vi "RPC Method Template.vi"(8 "error in (no error)":errorcluster, 11 "OOP Server in":refnum<class "OOP Query Server.lvclass">) -> (0 "error out":errorcluster)   [LabVIEW 2019, in "OOP Query Server.lvlib" / "OOP Query Server.lvclass"]
uses:
  OOP Query Server.lvclass
  OOP Query Server.lvclass/OOP Query Server.ctl
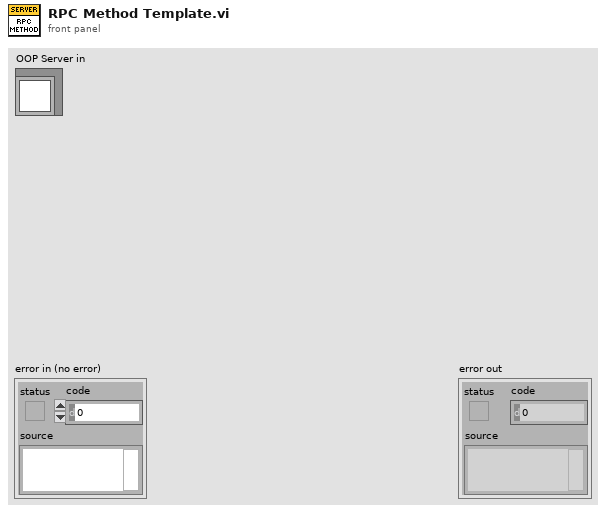
[diagram p1: front panel]
types:
  T1 = typedef "OOP Query Server.lvlib/OOP Query Server.lvclass/Server Internal UEs.ctl" = cluster{"Invoke Internal UE":refnum<user-event>, "Query Internal UE":refnum<user-event>, "Register Internal UE":refnum<user-event>}
  T2 = typedef "OOP Query Server.lvlib/OOP Query Server.lvclass/Server gRPC UEs.ctl" = cluster{"Invoke gRPC UE":refnum<user-event>, "Query gRPC UE":refnum<user-event>, "Register gRPC UE":refnum<user-event>}
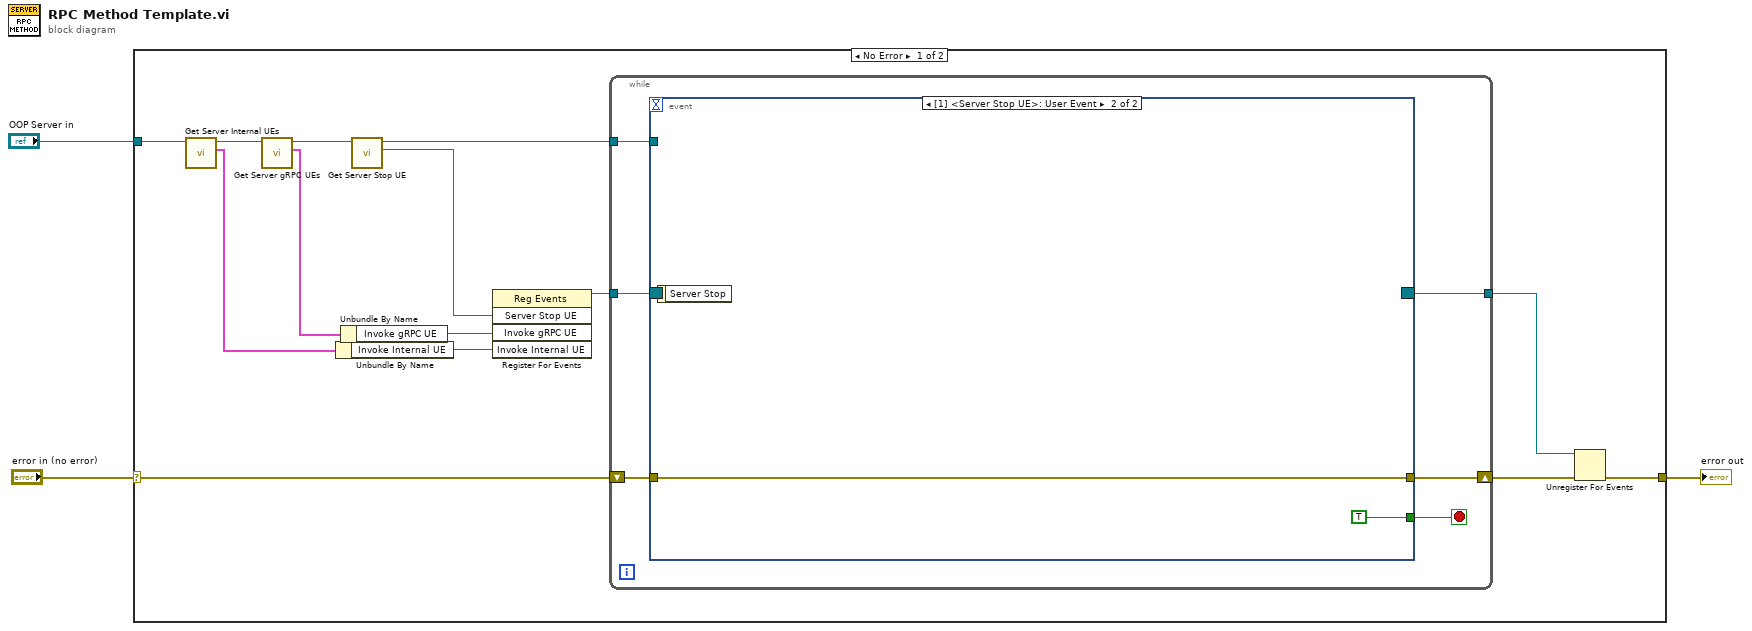
[diagram p0: block diagram]
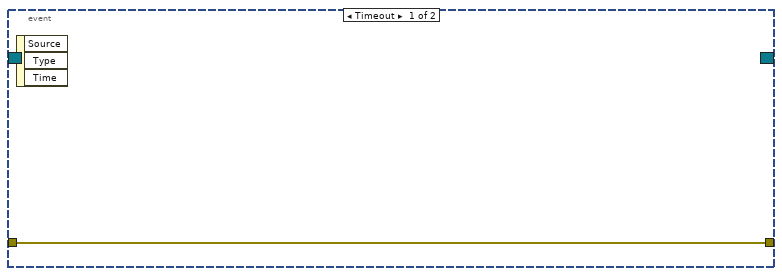
[diagram p2: hidden frame]
diagram:
  n1 = case shown="No Error" "error in (no error)" {
    selector: "error in (no error)" -> [w12 w27]
    tunnel: [w10 w27] -> w2
    tunnel: "OOP Server in" -> [w14 _]
    frame No Error {
      n2 = call "Get Server Internal UEs.vi"("OOP Server in"=w14) -> ("Server Internal UEs"=w6:T1, "OOP Server out"=w13:refnum<class "OOP Query Server.lvclass">)  [unwired: 9 in]
      n3 = call "Get Server gRPC UEs.vi"("OOP Server in"=w13) -> ("Server gRPC UEs"=w8:T2, "OOP Server out"=w17:refnum<class "OOP Query Server.lvclass">)  [unwired: 9 in]
      n4 = Unbundle By Name ("Unbundle Internal UE")(w6) -> ("Invoke Internal UE"=w5:refnum<user-event>)
      n5 = Unbundle By Name ("Unbundle gRPC UE")(w8) -> ("Invoke gRPC UE"=w7:refnum<user-event>)
      n6 = call "Get Server Stop UE.vi"("OOP Server in"=w17) -> ("Server Stop UE"=w16:refnum<user-event>, "OOP Server out"=w4:refnum<class "OOP Query Server.lvclass">)  [unwired: 9 in]
      n7 = register-events(w16, w7, w5) -> (reference out=w15:refnum<event-registration>)  [unwired: 2 in, 1 out]
      n8 = while {
        tunnel: w15 -> [w23]
        tunnel: [w19] -> w9
        shift-right: [w20] -> w11
        shift-left: w12 -> [w21]
        tunnel: w4 -> [w18]
        stop <- w22 stop-if-true
        n9 = event "RPC Method Event Structure" shown="[1] <Server Stop UE>: User Event" {
          selector: w23 -> [_ _]
          dyn-events: [_ _] -> w19
          timeout: _ -> [_ _]
          tunnel: [_ TRUE] -> w22
          tunnel: w21 -> [w24 w25]
          tunnel: [w24 w25] -> w20
          tunnel: w18 -> [_ _]
          event Timeout {
            n10 = event-data() -> ()  [unwired: 1 in, 3 out]
          }
          event User Event {
            n11 = event-data() -> ()  [unwired: 1 in, 1 out]
          }
        }
      }
      n12 = Unregister For Events(event registration refnum=w9, error in=w11) -> (error out=w10:errorcluster)
    }
    frame Error {
    }
  }
  "error out" <- w2
